vi "Parse Sensor Group 4.vi"(11 "stream in":u8[](array[numeric])) -> (1 "Sensor Group 4":T1, 3 "stream out":u8[](array[numeric]))   [LabVIEW 2014]
doc: "Read Sensor Group 4 from a UART data stream."
uses:
  Sensor Group 4.ctl
  Cargo Bay Digital Inputs.ctl
  Charging Sources Available.ctl
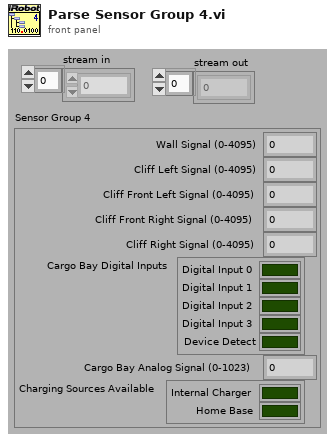
[diagram p1: front panel]
types:
  T1 = typedef "Sensor Group 4.ctl" = cluster{"Wall Signal (0-4095)":u16, "Cliff Left Signal (0-4095)":u16, "Cliff Front Left Signal (0-4095)":u16, "Cliff Front Right Signal (0-4095)":u16, "Cliff Right Signal (0-4095)":u16, "Cargo Bay Digital Inputs":T2, "Cargo Bay Analog Signal (0-1023)":u16, "Charging Sources Available":T3}
  T2 = typedef "Cargo Bay Digital Inputs.ctl" = cluster{"Digital Input 0":bool, "Digital Input 1":bool, "Digital Input 2":bool, "Digital Input 3":bool, "Device Detect":bool}
  T3 = typedef "Charging Sources Available.ctl" = cluster{"Internal Charger":bool, "Home Base":bool}
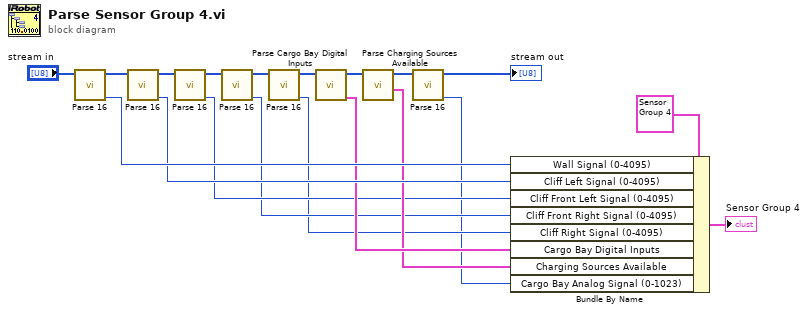
[diagram p0: block diagram]
diagram:
  n1 = call "Parse 16.vi"("stream in"="stream in") -> ("value"=w16:u16, "stream out"=w15:u8[])  [unwired: 9 out]
  n2 = call "Parse 16.vi"("stream in"=w15) -> ("value"=w14:u16, "stream out"=w13:u8[])  [unwired: 9 out]
  n3 = call "Parse 16.vi"("stream in"=w13) -> ("value"=w8:u16, "stream out"=w12:u8[])  [unwired: 9 out]
  n4 = call "Parse 16.vi"("stream in"=w12) -> ("value"=w7:u16, "stream out"=w6:u8[])  [unwired: 9 out]
  n5 = call "Parse 16.vi"("stream in"=w6) -> ("value"=w4:u16, "stream out"=w5:u8[])  [unwired: 9 out]
  n6 = call "Parse Cargo Bay Digital Inputs.vi"("stream in"=w5) -> ("Cargo Bay Digital Inputs"=w11:T2, "stream out"=w10:u8[])  [unwired: 9 out]
  n7 = call "Parse Charging Sources Available.vi"("stream in"=w10) -> ("Charging Sources Available"=w9:T3, "stream out"=w3:u8[])  [unwired: 9 out]
  n8 = call "Parse 16.vi"("stream in"=w3) -> ("value"=w2:u16, "stream out"=→"stream out":u8[])  [unwired: 9 out]
  n9 = Bundle By Name(cluster=T1 {"Wall Signal (0-4095)"=0, "Cliff Left Signal (0-4095)"=0, "Cliff Front Left Signal (0-4095)"=0, "Cliff Front Right Signal (0-4095)"=0, "Cliff Right Signal (0-4095)"=0, "Cargo Bay Digital Inputs"={"Digital Input 0"=FALSE, "Digital Input 1"=FALSE, "Digital Input 2"=FALSE, "Digital Input 3"=FALSE, "Device Detect"=FALSE}, "Cargo Bay Analog Signal (0-1023)"=0, "Charging Sources Available"={"Internal Charger"=FALSE, "Home Base"=FALSE}} ("Sensor Group 4"), "Wall Signal (0-4095)"=w16, "Cliff Left Signal (0-4095)"=w14, "Cliff Front Left Signal (0-4095)"=w8, "Cliff Front Right Signal (0-4095)"=w7, "Cliff Right Signal (0-4095)"=w4, "Cargo Bay Digital Inputs"=w11, "Charging Sources Available"=w9, "Cargo Bay Analog Signal (0-1023)"=w2) -> (→"Sensor Group 4":T1)
